vi "Report Firmware.vi"(8 "error in (no error)":errorcluster, 11 "Refnum In":refnum<vi>) -> (0 "error out":errorcluster, 1 "FirmataFirmwareVersion":string, 2 "FirmataFirmwareName":string, 3 "Refnum Out":refnum<vi>)   [LabVIEW 2020, in "FirmataClient.lvlib"]
doc: "Request the firmware name and version running on the target board."
uses:
  FirmataClient.lvlib
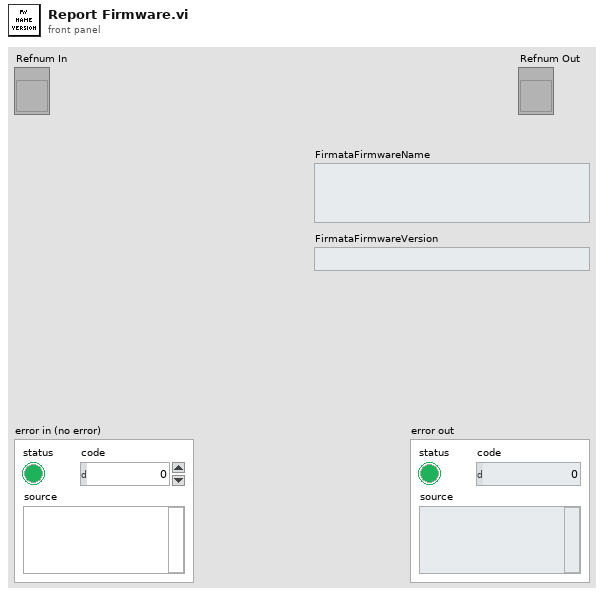
[diagram p1: front panel]
types:
  T1 = typedef "FirmataClient.lvlib/FirmataProtocolConstants.ctl" = u16
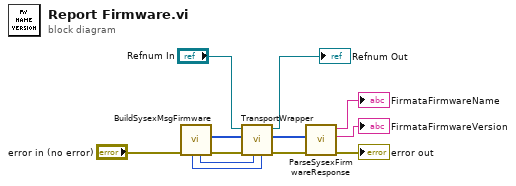
[diagram p0: block diagram]
diagram:
  n1 = call "BuildSysexMsgFirmware.vi"("error in"="error in (no error)") -> ("error out"=w10:errorcluster, "GetFirmwareMessage"=w2:u8[], "ReplyFirstByte"=w4:T1, "ReplyLength"=w3:i32)  [unwired: 7 in]
  n2 = call "TransportWrapper.vi"("ReplyLength"=w3, "ReplyFirstByte"=w4, "error in"=w10, "Message In"=w2, "Refnum In"="Refnum In") -> ("error out"=w12:errorcluster, "Message Out"=w1:u8[], "Refnum Out"=→"Refnum Out":refnum<vi>)  [unwired: 4 in]
  n3 = call "ParseSysexFirmwareResponse.vi"("error in"=w12, "Sysex Message"=w1) -> ("error out"=→"error out":errorcluster, "FirmataFirmwareVersion"=→"FirmataFirmwareVersion":string, "FirmataFirmwareName"=→"FirmataFirmwareName":string)  [unwired: 6 in, 1 out]
